vi "Set Switching.vi"(7 "measure call context in":refnum<class "Measure Call Context.lvclass">, 8 "error in":errorcluster, 11 "File Path":path) -> (0 "error out":errorcluster, 5 "measure call context out":refnum<class "Measure Call Context.lvclass">)   [LabVIEW 2023]
uses:
  Switch Settings.ctl
  <instrlib>/niSwitch/niSwitch.llb/niSwitch Path Capability.ctl
  <vilib>/Utility/file.llb/Read Delimited Spreadsheet (string).vi
  <instrlib>/niSwitch/niSwitch.llb/niSwitch Connect Channels (Single).vi
  <vilib>/ErrorRing/Error Ring.xnode
  <vilib>/Plug-In SDKs/Measurements/Measure Call Context/Measure Call Context.lvclass
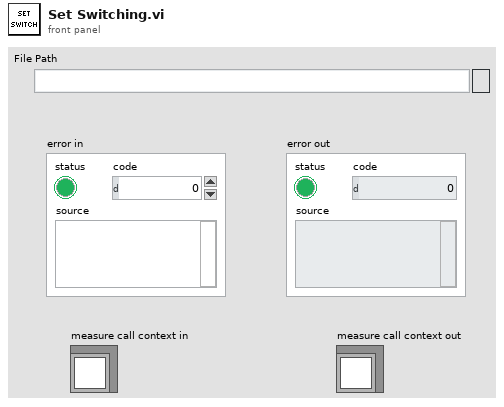
[diagram p1: front panel]
types:
  T1 = typedef "Switch Settings.ctl" = cluster{"Resource Name":refnum<k15>, "Channel 1":string, "Channel 2":string}
  T2 = typedef "niSwitch Path Capability.ctl" = i32
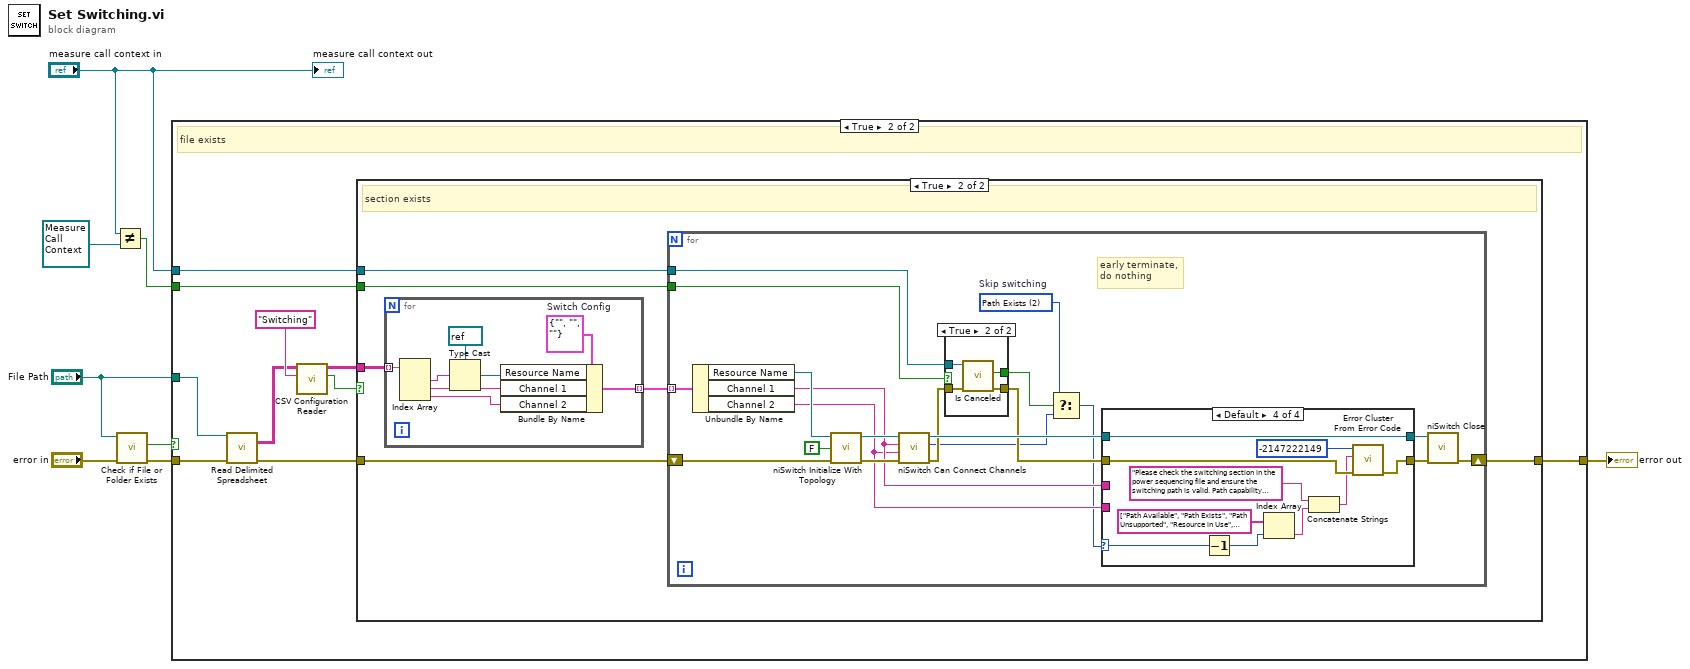
[diagram p0: block diagram]
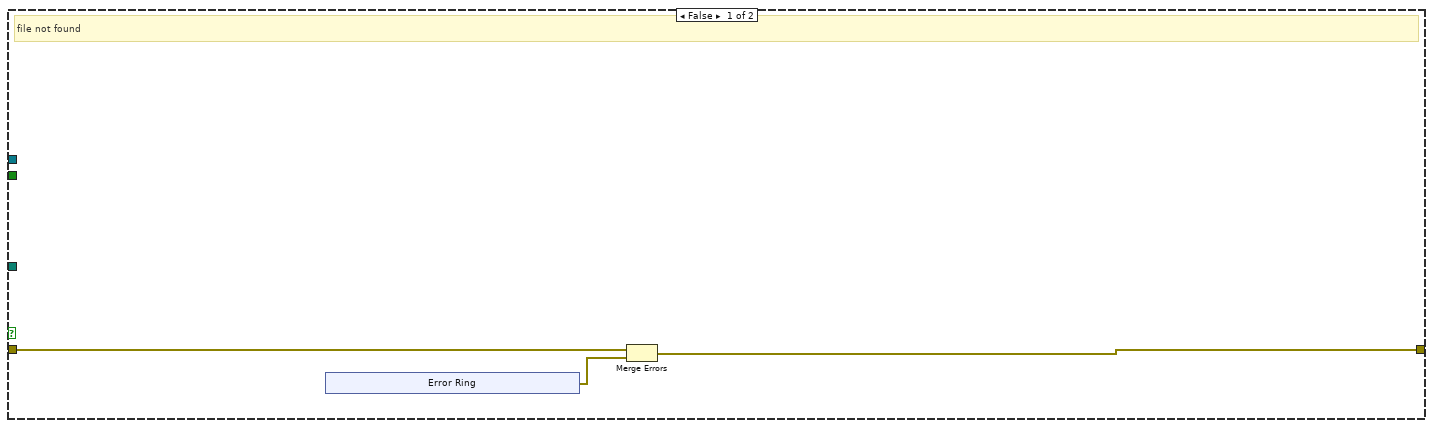
[diagram p2: hidden frame]
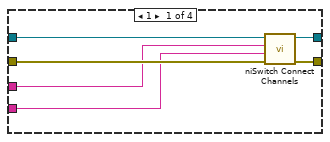
[diagram p5: hidden frame]
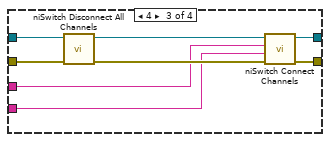
[diagram p7: hidden frame]
diagram:
  n1 = Not Equal?(x="measure call context in", y=refnum<class "Measure Call Context.lvclass"> refnum ("measure call context in")) -> (x != y?=w3:bool)
  n2 = call <vilib>:"Check if File or Folder Exists.vi"("error in (no error)"="error in", "path"="File Path") -> ("error out"=w5:errorcluster, "file or folder exists?"=w7:bool)  [unwired: 7 in, 1 out]
  n3 = case shown="True" w7 {
    tunnel: "File Path" -> [_ w25]
    tunnel: [w11 w21] -> w4
    tunnel: w5 -> [w10 w20]
    tunnel: "measure call context in" -> [_ w17]
    tunnel: w3 -> [_ w16]
    frame False {
      # "file not found"
      n4 = xnode "Error Ring"() -> ("error out"=w9:errorcluster)
      n5 = Merge Errors(w10, w9) -> (w11:errorcluster)
    }
    frame True {
      # "file exists"
      n6 = call-poly <vilib>:"Read Delimited Spreadsheet.vi"("file path (dialog if empty)"=w25, "error in (no error)"=w20) -> ("all rows"=w23:string[][], "error out"=w19:errorcluster)  [unwired: 8 in, 4 out]
      n7 = call "CSV Configuration Reader.vi"("Section"="Switching" ("element"), "All CSV Configurations"=w23) -> ("Section Exists?"=w18:bool, "Extracted Configurations"=w22:string[][])  [unwired: 8 in]
      n8 = case shown="True" w18 {
        tunnel: w22 -> [_ w32]
        tunnel: [w26 w30] -> w21
        tunnel: w19 -> [w26 w29]
        tunnel: w17 -> [_ w28]
        tunnel: w16 -> [_ w27]
        frame False {
          # "section not found, no switching required"
        }
        frame True {
          # "section exists"
          n9 = for {
            tunnel: w32 -> [w91] mode=indexing
            tunnel: [w88] -> w31 mode=indexing
            w84 = T1 {"Resource Name"="", "Channel 1"="", "Channel 2"=""}  # Switch Config
            n10 = Index Array(array=w91) -> (element #1=w90:string, element #2=w86:string, element #3=w85:string)  [unwired: 3 in]
            n11 = Type Cast(type=refnum<k15> refnum ("Resource Name"), x=w90) -> (*(type *) &x=w87:refnum<k15>)
            n12 = Bundle By Name(cluster=w84, "Resource Name"=w87, "Channel 1"=w86, "Channel 2"=w85) -> (w88:T1)
          }
          n13 = for {
            tunnel: w31 -> [w46] mode=indexing
            shift-right: [w42] -> w30
            shift-left: w29 -> [w41]
            tunnel: w28 -> [w38]
            tunnel: w27 -> [w33]
            w34 = T2 2 items=["Path Available"=1, "Path Exists"=2, "Path Unsupported"=3, "Resource in Use"=4, "Source Conflict"=5, "Channel Not Available"=6]  # Skip switching
            # "early terminate,\ndo nothing"
            n14 = Unbundle By Name(w46) -> ("Resource Name"=w45:refnum<k15>, "Channel 1"=w44:string, "Channel 2"=w43:string)
            n15 = call <instrlib>:"niSwitch Initialize With Topology.vi"("error in (no error)"=w41, "reset device (boolean value)"=FALSE, "resource name"=w45) -> ("error out"=w51:errorcluster, "instrument handle out"=w52:refnum<k15>)  [unwired: 7 in]
            n16 = call <instrlib>:"niSwitch Can Connect Channels.vi"("error in (no error)"=w51, "channel 2"=w43, "channel 1"=w44, "instrument handle"=w52) -> ("error out"=w40:errorcluster, "path capability"=w36:T2, "instrument handle out"=w49:refnum<k15>)  [unwired: 5 in]
            n17 = case shown="True" w33 {
              tunnel: w40 -> [w53 w57]
              tunnel: [w53 w56] -> w39
              tunnel: w38 -> [_ w55]
              tunnel: [_ w54] -> w37
              frame False {
              }
              frame True {
                n18 = call <vilib>:"Is Canceled.vi"("error in"=w57, "measure call context in"=w55) -> ("error out"=w56:errorcluster, "is canceled?"=w54:bool)  [unwired: 7 in, 1 out]
              }
            }
            n19 = Select(t=w34, s=w37, f=w36) -> (s? t:f=w35:T2)
            n20 = case shown="Default" w35 {
              selector: w35 -> [_ _ _ w75]
              tunnel: w49 -> [w63 w65 w73 w83]
              tunnel: w39 -> [w62 w64 w72 w82]
              tunnel: w43 -> [w61 _ w70 _]
              tunnel: w44 -> [w60 _ w69 _]
              tunnel: [w59 w65 w67 w83] -> w47
              tunnel: [w58 w64 w66 w81] -> w48
              frame 1 {
                n21 = call-poly <instrlib>:"niSwitch Connect Channels.vi"("error in (no error)"=w62, "channel 2"=w61, "channel 1"=w60, "instrument handle"=w63) -> ("error out"=w58:errorcluster, "instrument handle out"=w59:refnum<k15>)  [unwired: 6 in]
              }
              frame 2 {
              }
              frame 4 {
                n22 = call <instrlib>:"niSwitch Disconnect All Channels.vi"("error in (no error)"=w72, "instrument handle"=w73) -> ("error out"=w71:errorcluster, "instrument handle out"=w68:refnum<k15>)  [unwired: 8 in]
                n23 = call-poly <instrlib>:"niSwitch Connect Channels.vi"("error in (no error)"=w71, "channel 2"=w70, "channel 1"=w69, "instrument handle"=w68) -> ("error out"=w66:errorcluster, "instrument handle out"=w67:refnum<k15>)  [unwired: 6 in]
              }
              frame Default {
                n24 = Decrement(x=w75) -> (x-1=w74:T2)
                n25 = Index Array(array=string[] ["Path Available", "Path Exists", "Path Unsupported", "Resource in Use", "Source Conflict", "Channel Not Available"] ("Strings []"), index=w74) -> (element=w76:string)
                n26 = Concatenate Strings("Please check the switching section in the power sequencing file and ensure the switching path is valid. Path capability error: ", w76) -> (w78:string)
                n27 = call <vilib>:"Error Cluster From Error Code.vi"("error in (no error)"=w82, "error message (\"\")"=w78, "error code (0)"=-2147222149) -> ("error out"=w81:errorcluster)  [unwired: 6 in]
              }
            }
            n28 = call <instrlib>:"niSwitch Close.vi"("error in (no error)"=w48, "instrument handle"=w47) -> ("error out"=w42:errorcluster)  [unwired: 9 in]
          }
        }
      }
    }
  }
  "error out" <- w4
  "measure call context out" <- "measure call context in"
